vi "New.vi"(6 "Unescape?":bool, 7 "Parent":refnum<class "NonTerminal.lvclass">, 8 "Error In":errorcluster, 11 "Key":string) -> (0 "Error Out":errorcluster, 3 "Tag":refnum<class "Tag.lvclass">)   [LabVIEW 2018, in "Toolkit.lvlib" / "Nodes.lvlib" / "Tag.lvclass"]
uses:
  Tag.lvclass
  NonTerminal/NonTerminal.lvclass
  D:/Users/cfield/Code/Field R&D Services/Mustache/trunk/src/Toolkit/Nodes/Abstract/Abstract.lvclass
  Tag.lvclass/Tag.ctl
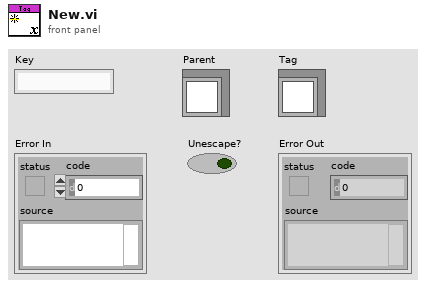
[diagram p1: front panel]
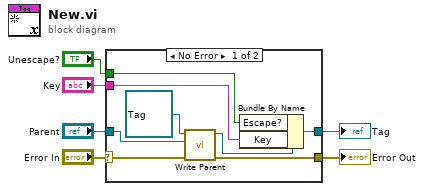
[diagram p0: block diagram]
diagram:
  n1 = case shown="No Error" "Error In" {
    selector: "Error In" -> [w10 w15]
    tunnel: [w9 w15] -> w6
    tunnel: "Key" -> [w13 _]
    tunnel: [w14 _] -> w2
    tunnel: "Parent" -> [w11 _]
    tunnel: "Unescape?" -> [w7 _]
    frame No Error {
      n2 = call-dynamic "Write Parent.vi"("Error In"=w10, "Parent"=w11, "Node In"=refnum<class "Tag.lvclass"> refnum ("Toolkit.lvlib:Nodes.lvlib:EscapedTag.lvclass")) -> ("Error Out"=w9:errorcluster, "Node Out"=w8:refnum<class "Tag.lvclass">)  [unwired: 7 in]
      n3 = Bundle By Name(cluster=w8, "Escape?"=w7, "Key"=w13) -> (w14:refnum<class "Tag.lvclass">)
    }
    frame Error {
    }
  }
  "Error Out" <- w6
  "Tag" <- w2
